vi "Library Name.vi"() -> (3 "library name":string)   [LabVIEW 2017, in "DSF Core.lvlib" / "DSF UDP Transceiver.lvclass"]
uses:
  DSF UDP Transceiver.lvclass
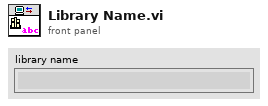
[diagram p1: front panel]
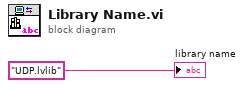
[diagram p0: block diagram]
diagram:
  "library name" <- "UDP.lvlib" ("base error code")
